vi "ReadArraySingle(SGL).vi"(8 "error in (no error)":errorcluster, 9 "Elements (-1 = auto)":i32=-1, 10 "variableName":string, 11 "TCatAdsNet in":refnum<class "AdsNET.lvclass">) -> (0 "error out":errorcluster, 1 "Elements":i32, 2 "Values (SGL)":sgl[](array[numeric]), 3 "TCatAdsNet out":refnum<class "AdsNET.lvclass">, 4 "Elapsed Time (ms)":u32)   [LabVIEW 2016, in "TCatAdsNet.lvlib" / "AdsNET.lvclass"]
uses:
  AdsNET.lvclass
  AdsNET.lvclass/AdsNET.ctl
  C:/Users/Maurizio/Projects/sentiero-beckoff/DLL/TwinCAT.Ads.dll
  sentiero-beckoff/DLL/TwinCAT.Ads.dll
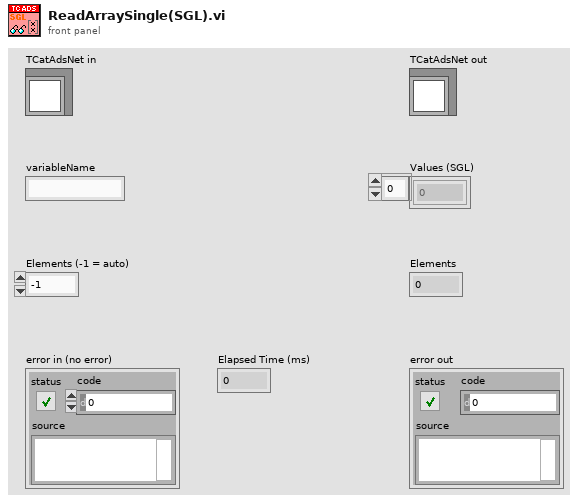
[diagram p1: front panel]
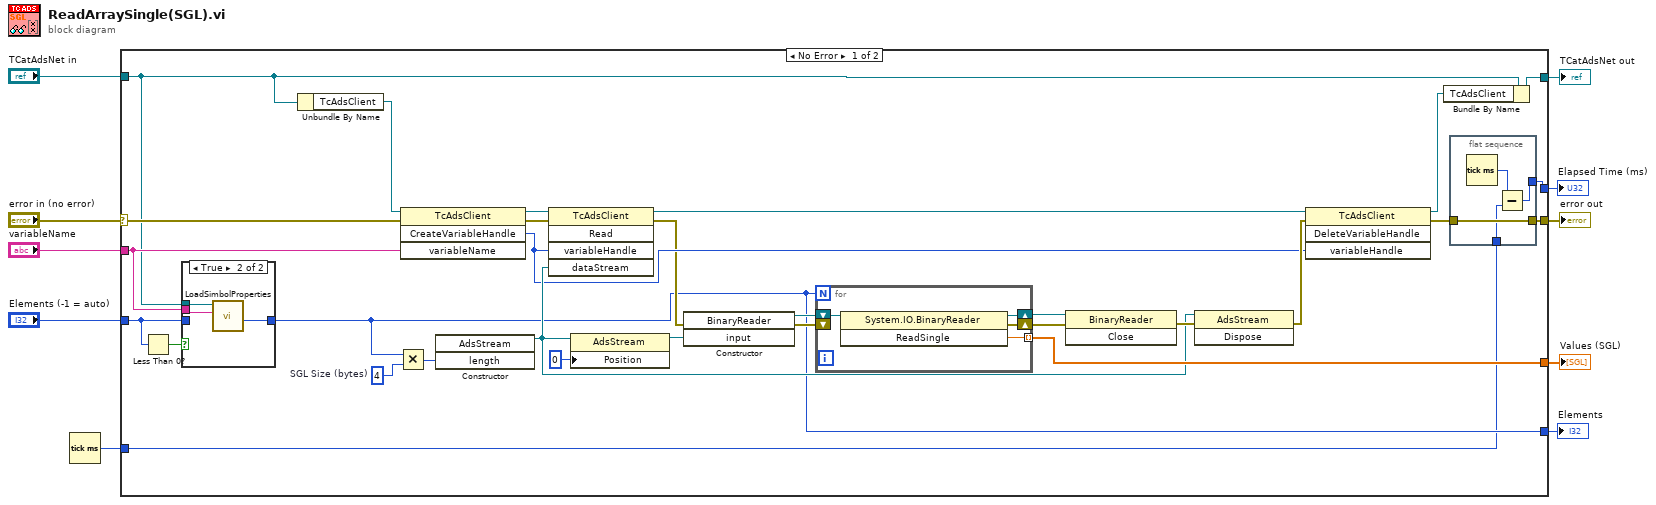
[diagram p0: block diagram]
diagram:
  n1 = Tick Count (ms)() -> (millisecond timer value=w2:u32)
  n2 = case shown="No Error" "error in (no error)" {
    selector: "error in (no error)" -> [w20 w53]
    tunnel: [w33 _] -> w10
    tunnel: "variableName" -> [w16 _]
    tunnel: "Elements (-1 = auto)" -> [w18 _]
    tunnel: [w22 w54] -> w7
    tunnel: [w14 w53] -> w6
    tunnel: "TCatAdsNet in" -> [w15 w54]
    tunnel: [w17 _] -> w3
    tunnel: w2 -> [w12 _]
    tunnel: [w11 _] -> w1
    frame No Error {
      w38 = 4  # SGL Size (bytes)
      n3 = Less Than 0?(x=w18) -> (x < 0?=w19:bool)
      n4 = case shown="True" w19 {
        tunnel: w18 -> [w45 _]
        tunnel: [w45 w48] -> w17
        tunnel: w15 -> [_ w47]
        tunnel: w16 -> [_ w46]
        frame False {
        }
        frame True {
          n5 = call "LoadSimbolProperties.vi"("name"=w46, "TCatAdsNet in"=w47) -> ("Elements"=w48:i32)  [unwired: 6 in, 3 out]
        }
      }
      n6 = Unbundle By Name(w15) -> ("TcAdsClient"=w23:refnum<k24>)
      n7 = Multiply ("Multiplizieren")(x=w17, y=w38) -> (x*y=w37:i32)
      n8 = invoke class="TcAdsClient" method="CreateVariableHandle"(reference=w23, error in=w20, "variableName"=w16) -> (reference out=w40:refnum<k24>, error out=w39:errorcluster, "CreateVariableHandle"=w25:i32)  [unwired: 1 in, 1 out]
      n9 = constructor class="AdsStream" ("Konstruktorknoten")("length"=w37) -> (reference out=w27:refnum<k24>)  [unwired: 3 in, 3 out]
      n10 = invoke class="TcAdsClient" method="Read"(reference=w40, error in=w39, "variableHandle"=w25, "dataStream"=w27) -> (reference out=w28:refnum<k24>, error out=w24:errorcluster)  [unwired: 1 in, 3 out]
      n11 = property class="AdsStream"(reference=w27, "Position"=i64 0) -> (reference out=w35:refnum<k24>)  [unwired: 1 in, 1 out]
      n12 = constructor class="BinaryReader"(error in=w24, "input"=w35) -> (reference out=w34:refnum<k24>, error out=w31:errorcluster)  [unwired: 2 in, 2 out]
      n13 = for {
        N: w17 -> [_]
        tunnel: [w51] -> w33 mode=indexing
        shift-right: [w50] -> w32
        shift-left: w34 -> [w52]
        shift-right: [w49] -> w30
        shift-left: w31 -> [_]
        n14 = invoke class="System.IO.BinaryReader" method="ReadSingle"(reference=w52) -> (reference out=w50:refnum<k24>, error out=w49:errorcluster, "ReadSingle"=w51:sgl)  [unwired: 2 in]
      }
      n15 = invoke class="BinaryReader" method="Close"(reference=w32, error in=w30) -> (error out=w29:errorcluster)  [unwired: 1 in, 2 out]
      n16 = invoke class="AdsStream" method="Dispose"(reference=w27, error in=w29) -> (error out=w26:errorcluster)  [unwired: 1 in, 2 out]
      n17 = invoke class="TcAdsClient" method="DeleteVariableHandle"(reference=w28, error in=w26, "variableHandle"=w25) -> (reference out=w21:refnum<k24>, error out=w13:errorcluster)  [unwired: 1 in, 2 out]
      n18 = Bundle By Name(cluster=w15, "TcAdsClient"=w21) -> (w22:refnum<class "AdsNET.lvclass">)
      n19 = flat-sequence {
        tunnel: [w44] -> w14
        tunnel: w13 -> [w44]
        tunnel: w12 -> [w42]
        tunnel: [w41] -> w11
        frame #0 {
          n20 = Tick Count (ms)() -> (millisecond timer value=w43:u32)
          n21 = Subtract(x=w43, y=w42) -> (x-y=w41:u32)
        }
      }
    }
    frame Error {
    }
  }
  "TCatAdsNet out" <- w7
  "Values (SGL)" <- w10
  "error out" <- w6
  "Elements" <- w3
  "Elapsed Time (ms)" <- w1
